vi "All Stations Part Config.vi"() -> ()   [LabVIEW 2018]
panel:
  in  "Exit Edit":bool
  in  "Add New Line":bool
  in  "精切":bool
  in  "Part Type":u16(ring) items=["V254"]
  in  "粗切":bool
  # "ALL Stations Recipe Config"
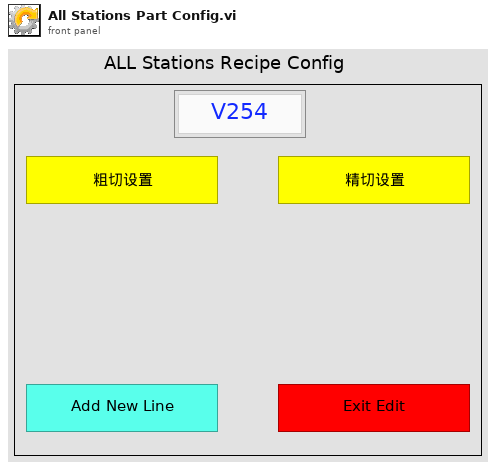
[diagram p1: front panel]
types:
  T1 = cluster{"station name":string, "line name":string, "Base path":path}
  T2 = enum16{"open", "replace", "create", "open or create", "replace or create", "replace or create with confirmation"}
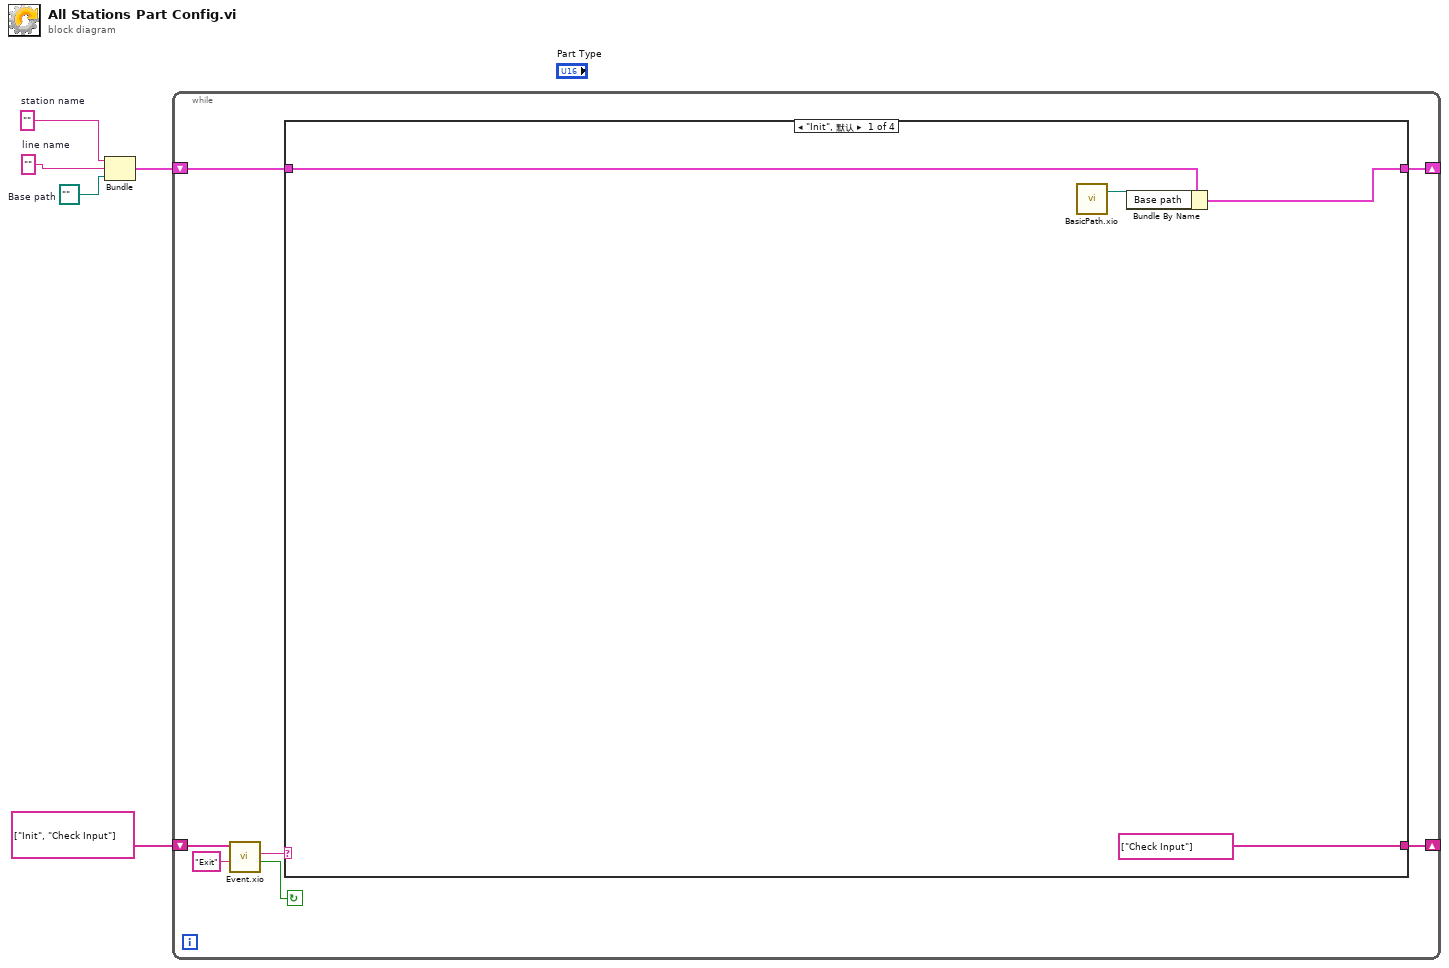
[diagram p0: block diagram]
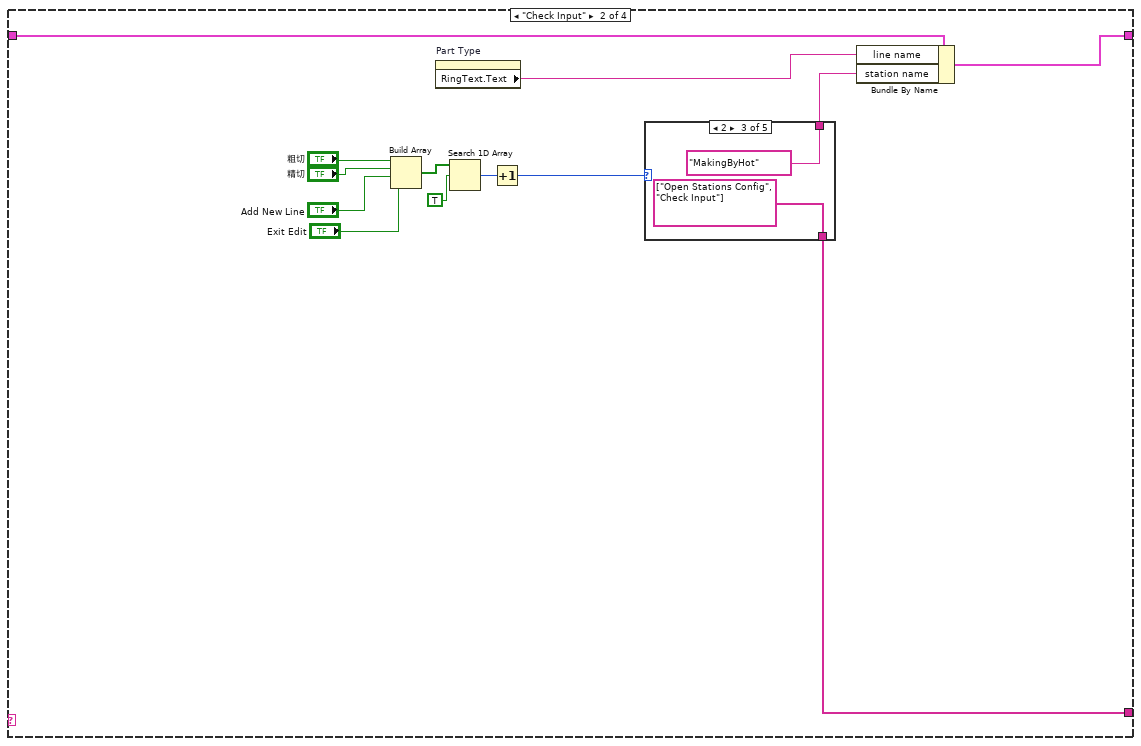
[diagram p2: hidden frame]
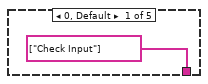
[diagram p3: hidden frame]
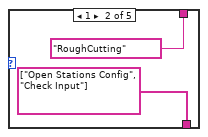
[diagram p4: hidden frame]
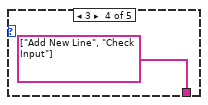
[diagram p5: hidden frame]
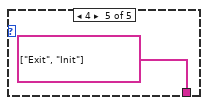
[diagram p6: hidden frame]
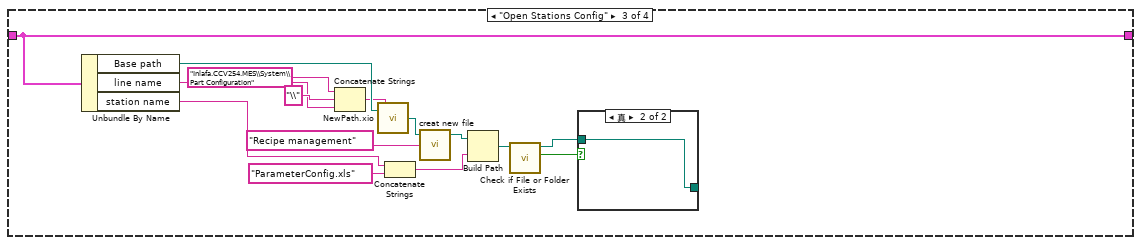
[diagram p7: hidden frame]
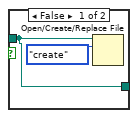
[diagram p8: hidden frame]
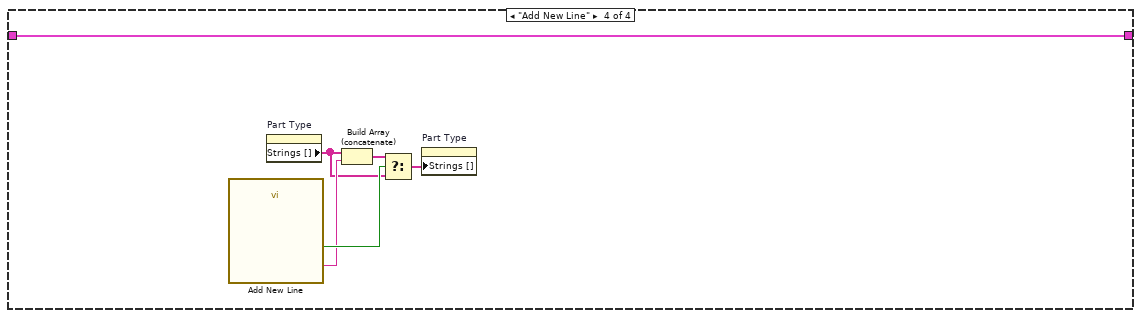
[diagram p9: hidden frame]
diagram:
  w1 = ""  # station name
  w2 = ""  # line name
  w3 = path ""  # Base path
  n1 = Bundle("station name"=w1, "line name"=w2, "Base path"=w3) -> (w4:T1)  [unwired: 1 in]
  n2 = while {
    shift-right: [w9] -> _
    shift-left: string[] ["Init", "Check Input"] -> [w11]
    shift-right: [w7] -> _
    shift-left: w4 -> [w8]
    stop <- w6 continue-if-true
    n3 = call "Event.xio.vi"("标志事件"="Exit", "事件组"=w11) -> ("？"=w6:bool, "下一事件"=w12:string)  [unwired: 3 in, 3 out]
    n4 = case shown="\"Init\", 默认" w12 {
      tunnel: [string[] ["Check Input"] w23 _ _] -> w9
      tunnel: w8 -> [w15 w22 w51 w56]
      tunnel: [w14 w21 w51 w56] -> w7
      frame "Init", Default {
        n5 = call "BasicPath.xio.vi"() -> ("stripped path"=w13:path)  [unwired: 1 in, 1 out]
        n6 = Bundle By Name(cluster=w15, "Base path"=w13) -> (w14:T1)
      }
      frame "Check Input" {
        n7 = Build Array("粗切", "精切", "Add New Line", "Exit Edit") -> (w27:bool[])
        n8 = property on="Part Type" class="Ring (严格)"() -> ("RingText.Text"=w18:string)  [unwired: 2 in, 2 out]
        n9 = Search 1D Array(1D array=w27, element=TRUE ("元素")) -> (index of element=w25:i32)  [unwired: 1 in]
        n10 = Increment(x=w25) -> (x+1=w24:i32)
        n11 = case shown="2" w24 {
          tunnel: [string[] ["Check Input"] string[] ["Open Stations Config", "Check Input"] string[] ["Open Stations Config", "Check Input"] string[] ["Add New Line", "Check Input"] string[] ["Exit", "Init"]] -> w23
          tunnel: [_ "RoughCutting" "MakingByHot" _ _] -> w20
          frame 0, Default {
          }
          frame 1 {
          }
          frame 2 {
          }
          frame 3 {
          }
          frame 4 {
          }
        }
        n12 = Bundle By Name(cluster=w22, "line name"=w18, "station name"=w20) -> (w21:T1)
      }
      frame "Open Stations Config" {
        n13 = Unbundle By Name(w51) -> ("Base path"=w50:path, "line name"=w47:string, "station name"=w37:string)
        n14 = Concatenate Strings("Inlafa.CCV254.MES\\System\\Part Configuration", "\\" ("字符串"), w47) -> (w46:string)
        n15 = call "NewPath.xio.vi"("Append path"=w46, "Basic path"=w50) -> ("New path"=w45:path)
        n16 = Concatenate Strings(w37, "ParameterConfig.xls" ("file name")) -> (w40:string)
        n17 = call "creat new file.vi"("file name"="Recipe management", "path"=w45) -> ("created path"=w43:path)  [unwired: 1 in, 2 out]
        n18 = Build Path(base path=w43, name or relative path=w40) -> (appended path=w42:path)
        n19 = call <vilib>:"Check if File or Folder Exists.vi"("path"=w42) -> ("file or folder exists?"=w39:bool, "dup path"=w38:path)  [unwired: 8 in, 1 out]
        n20 = case shown="真" w39 {
          tunnel: w38 -> [w52 w54]
          tunnel: [w52 w54] -> _
          frame False {
            n21 = Open/Create/Replace File(file path (use dialog)=w52, operation (0:open)=T2."create" ("操作(0:open)")) -> ()  [unwired: 4 in, 3 out]
          }
          frame True {
          }
        }
      }
      frame "Add New Line" {
        n22 = call "Add New Line"() -> ("产线名称"=w57:string, "确定"=w58:bool)  [unwired: 17 in, 1 out]
        n23 = property on="Part Type" class="Ring (严格)"() -> ("Strings []"=w55:string[])  [unwired: 2 in, 2 out]
        n24 = Build Array (concatenate)(w55, w57) -> (w60:string[])
        n25 = Select(t=w60, s=w58, f=w55) -> (s? t:f=w59:string[])
        n26 = property on="Part Type" class="Ring (严格)"("Strings []"=w59) -> ()  [unwired: 2 in, 2 out]
      }
    }
  }
